vi "meanAllMeaser (SubVI).vi"(10 "mMean":i32=64, 11 "MeasIn":T1 {"FFT amplitude mean" format="%.2p"; "DC" format="%0.2p"; "time trig 2" format="%0.2p"; "time trig" format="%0.2p"; "detected frequency 2" format="%.2p"; "way sensor 2" format="%.2p"; "way sensor 1" format="%.2p"; "detected frequency" format="%.2p"; "RMS" format="%0.2p"; "amplitude" format="%.2p"; "FFT amplitude" format="%.2p"}) -> (3 "MeasOut":T1 {"FFT amplitude mean" format="%.2p"; "DC" format="%0.2p"; "time trig 2" format="%0.2p"; "time trig" format="%0.2p"; "detected frequency 2" format="%.2p"; "way sensor 2" format="%.2p"; "way sensor 1" format="%.2p"; "detected frequency" format="%.2p"; "RMS" format="%0.2p"; "amplitude" format="%.2p"; "FFT amplitude" format="%.2p"})   [LabVIEW 2017]
uses:
  Control_EU/MeasControl.ctl
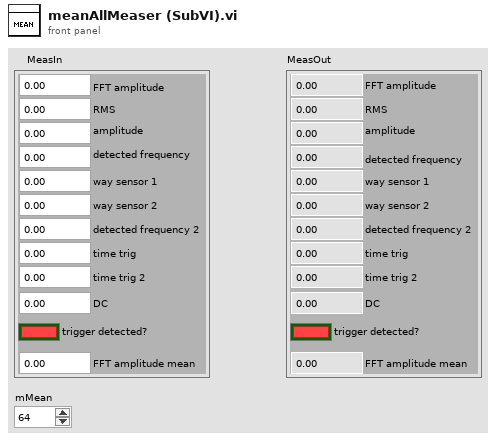
[diagram p1: front panel]
types:
  T1 = typedef "MeasControl.ctl" = cluster{"FFT amplitude":dbl, "amplitude":dbl, "RMS":dbl, "detected frequency":dbl, "way sensor 1":ext, "way sensor 2":ext, "detected frequency 2":dbl, "time trig":dbl, "time trig 2":dbl, "DC":dbl, "trigger detected?":bool, "FFT amplitude mean":dbl}
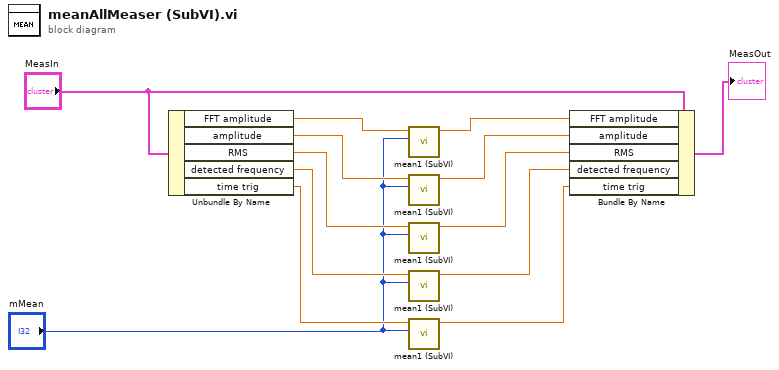
[diagram p0: block diagram]
diagram:
  n1 = Unbundle By Name("MeasIn") -> ("FFT amplitude"=w12:dbl, "amplitude"=w11:dbl, "RMS"=w10:dbl, "detected frequency"=w9:dbl, "time trig"=w3:dbl)
  n2 = call "mean1 (SubVI).vi"("mMean"="mMean", "detected amplitude"=w12) -> ("mean"=w8:dbl)  [unwired: 8 in, 1 out]
  n3 = call "mean1 (SubVI).vi"("mMean"="mMean", "detected amplitude"=w11) -> ("mean"=w7:dbl)  [unwired: 8 in, 1 out]
  n4 = call "mean1 (SubVI).vi"("mMean"="mMean", "detected amplitude"=w10) -> ("mean"=w6:dbl)  [unwired: 8 in, 1 out]
  n5 = call "mean1 (SubVI).vi"("mMean"="mMean", "detected amplitude"=w9) -> ("mean"=w5:dbl)  [unwired: 8 in, 1 out]
  n6 = call "mean1 (SubVI).vi"("mMean"="mMean", "detected amplitude"=w3) -> ("mean"=w2:dbl)  [unwired: 8 in, 1 out]
  n7 = Bundle By Name(cluster="MeasIn", "FFT amplitude"=w8, "amplitude"=w7, "RMS"=w6, "detected frequency"=w5, "time trig"=w2) -> (→"MeasOut":T1)
